vi "CODMN外部API.vi"() -> ()   [LabVIEW 2016, in "斯坦道CODMn.lvlib"]
panel:
  out "配置文件 path":path
  out "ping":bool
  out "CODMn状态":u16(ring) caption="氨氮状态" items=["待机", "润洗", "进样", "进样完成", "柱塞泵加标", "等待取液", "排液"]
  out "远程反控校零CODMn":bool
  out "远程反控校准CODMn":bool
  out "手动启动CODMn":bool
  in  "自动切换量程":bool=TRUE
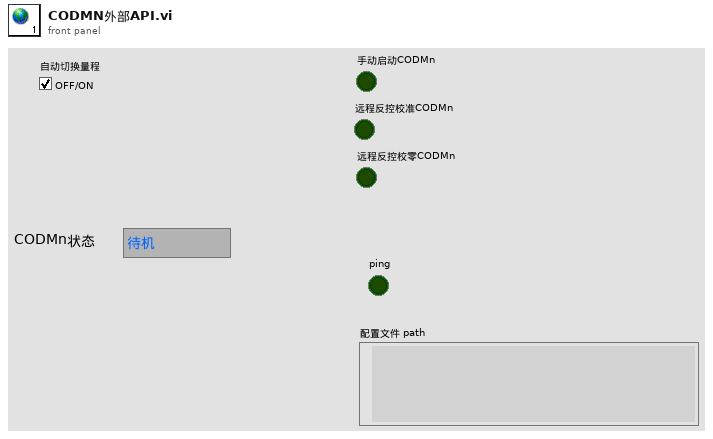
[diagram p1: front panel]
diagram:
